vi "Empty VCluster Constant__ogtk.vi"() -> (0 "Empty Cluster":variant)   [LabVIEW 2023, in "openg_variant.lvlib"]
uses:
  openg_variant.lvlib
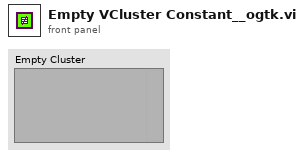
[diagram p1: front panel]
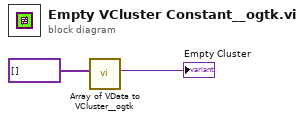
[diagram p0: block diagram]
diagram:
  n1 = call "Array of VData to VCluster__ogtk.vi"("Array"=variant[] []) -> ("VCluster"=→"Empty Cluster":variant)  [unwired: 9 in, 1 out]
